vi "Execute.vi"(10 "Test Runner V2 in":refnum<class "Runnable.lvclass">, 11 "Single Thread Test Runner In":refnum<class "Single Thread Test Runner.lvclass">) -> ()   [LabVIEW 2020, in "Single Thread Test Runner.lvclass"]
uses:
  Single Thread Test Runner.lvclass
  Core/Runnable/Runnable.lvclass
  Single Thread Test Runner.lvclass/Single Thread Test Runner.ctl
  Result Observer/Result Observer.lvclass
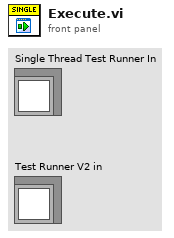
[diagram p1: front panel]
types:
  T1 = typedef "Result.lvlib/Result.ctl" = cluster{"Name":string, "Message":string, "Description":string, "Status":T2, "Result Type":T3, "Execution Time":dbl}
  T2 = typedef "Result.lvlib/Status.ctl" = enum16{"", "Passed", "Failed", "Error", "Skipped", "Setup Error", "Broken", "Teardown Error"}
  T3 = typedef "Result.lvlib/Type.ctl" = enum16{"Test Case", "Test Suite", "Test Run", "Pass", "Fail", "Skip", "Pass if", "Fail if", "Pass if Error", "Fail if Error", "Pass if Equal", "Fail if Equal"}
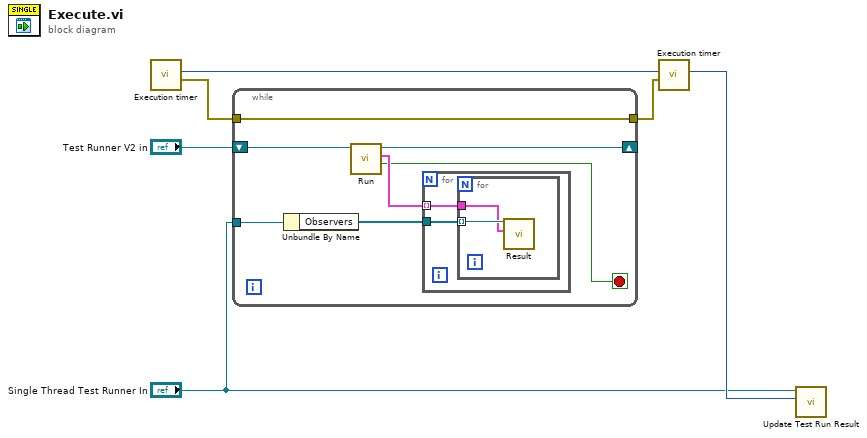
[diagram p0: block diagram]
diagram:
  n1 = call "Execution timer.vi"() -> ("error out"=w1:errorcluster, "Current or Duration [ms]"=w5:u32)  [unwired: 10 in]
  n2 = while {
    shift-right: [w11] -> _
    shift-left: "Test Runner V2 in" -> [w13]
    tunnel: "Single Thread Test Runner In" -> [w10]
    tunnel: [w7] -> w2
    tunnel: w1 -> [w7]
    stop <- w9 stop-if-true
    n3 = Unbundle By Name(w10) -> ("Observers"=w8:refnum<class "Result Observer.lvclass">[])
    n4 = call-dynamic "Run.vi"("Runnable In"=w13) -> ("Done?"=w9:bool, "Results"=w12:T1[], "Runnable Out"=w11:refnum<class "Runnable.lvclass">)  [unwired: 7 in, 1 out]
    n5 = for {
      tunnel: w12 -> [w14] mode=indexing
      tunnel: w8 -> [w15]
      n6 = for {
        tunnel: w15 -> [w17] mode=indexing
        tunnel: w14 -> [w16]
        n7 = call-dynamic "Result.vi"("Result"=w16, "Result Observer In"=w17) -> ()  [unwired: 9 in, 1 out]
      }
    }
  }
  n8 = call "Execution timer.vi"("error in (no error)"=w2, "millisecond timer value"=w5) -> ("Current or Duration [ms]"=w4:u32)  [unwired: 8 in, 1 out]
  n9 = call "Update Test Run Result.vi"("Duration [ms]"=w4, "Single Thread Test Runner in"="Single Thread Test Runner In") -> ()  [unwired: 9 in, 1 out]
